vi "Write K_i.vi"(8 "error in (no error)":errorcluster, 10 "K_i":dbl, 11 "Altitude Guidance in":refnum<class "Altitude Guidance.lvclass">) -> (0 "error out":errorcluster, 3 "Altitude Guidance out":refnum<class "Altitude Guidance.lvclass">)   [LabVIEW 2014, in "Guidance Library.lvlib" / "Altitude Guidance.lvclass"]
uses:
  Altitude Guidance.lvclass
  Altitude Guidance.lvclass/Altitude Guidance.ctl
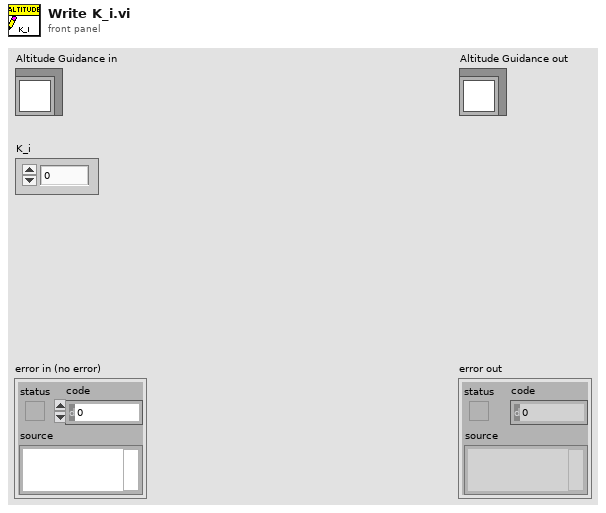
[diagram p1: front panel]
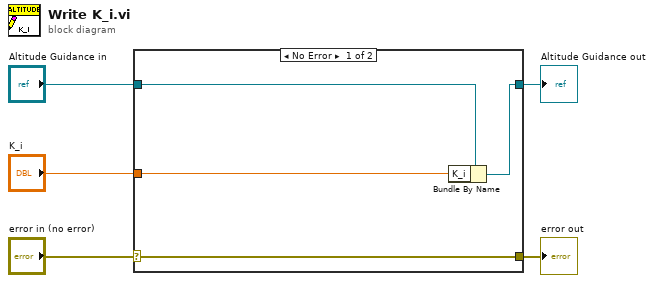
[diagram p0: block diagram]
diagram:
  n1 = case shown="No Error" "error in (no error)" {
    selector: "error in (no error)" -> [w9 w10]
    tunnel: [w9 w10] -> w4
    tunnel: [w7 w11] -> w2
    tunnel: "Altitude Guidance in" -> [w8 w11]
    tunnel: "K_i" -> [w6 _]
    frame No Error {
      n2 = Bundle By Name(cluster=w8, "K_i"=w6) -> (w7:refnum<class "Altitude Guidance.lvclass">)
    }
    frame Error {
    }
  }
  "error out" <- w4
  "Altitude Guidance out" <- w2
